vi "Init Device.vi"(8 "error in (no error)":errorcluster, 11 "Virtual Microscope in":refnum<class "Virtual Microscope.lvclass">) -> (0 "error out":errorcluster, 3 "Virtual Microscope out":refnum<class "Virtual Microscope.lvclass">)   [LabVIEW 2015, in "Virtual Microscope.lvlib" / "Virtual Microscope.lvclass"]
uses:
  Virtual Microscope.lvclass
  Virtual Microscope.lvclass/Virtual Microscope.ctl
  TE2000/TE2000.lvclass
  Eclipse TI/Eclipse TI.lvclass
  Device/Device.lvclass
  <vilib>/ActorFramework/Actor/Actor.lvclass
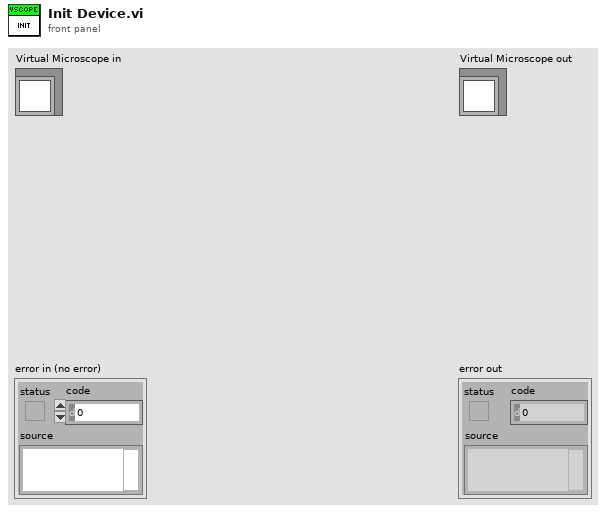
[diagram p1: front panel]
types:
  T1 = typedef "Microscope Configuration.ctl" = cluster{"Serial Port":refnum<visa-resource-name>, "Microscope Type":T2, "FilterBlockCassette1":refnum<k7>, "LightPathDrive":refnum<k7>, "INikonTI":refnum<k7>}
  T2 = typedef "Microscope Type.ctl" = enum16{"TE2000", "Eclipse Ti"}
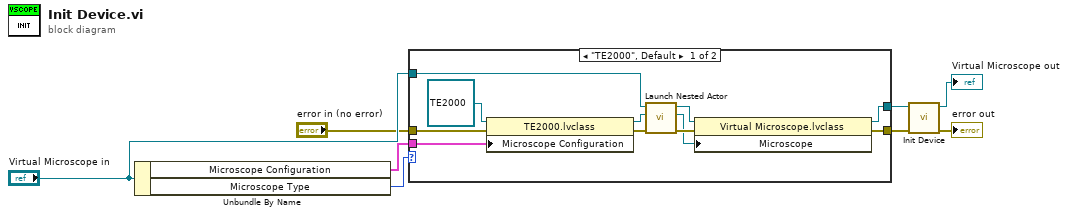
[diagram p0: block diagram]
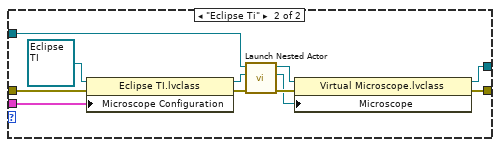
[diagram p2: hidden frame]
diagram:
  n1 = Unbundle By Name("Virtual Microscope in") -> ("Microscope Configuration"=w6:T1, "Microscope Type"=w5:T2)
  n2 = case shown="\"TE2000\", Default" w5 {
    tunnel: "Virtual Microscope in" -> [w18 w30]
    tunnel: [w12 w21] -> w1
    tunnel: w6 -> [w16 w28]
    tunnel: "error in (no error)" -> [w15 w27]
    tunnel: [w11 w23] -> w2
    frame "TE2000", Default {
      n3 = property class="TE2000.lvclass"(reference=refnum<class "TE2000.lvclass"> refnum ("TE2000.lvlib:TE2000.lvclass"), error in=w15, "Microscope Configuration"=w16) -> (reference out=w17:refnum<class "TE2000.lvclass">, error out=w14:errorcluster)
      n4 = call <vilib>:"Launch Nested Actor.vi"("error in (no error)"=w14, "Nested Actor"=w17, "Caller Actor in"=w18) -> ("error out"=w10:errorcluster, "Nested Actor's Enqueuer"=w9:refnum<class "Message Enqueuer.lvclass">, "Caller Actor out"=w13:refnum<class "Virtual Microscope.lvclass">)  [unwired: 6 in]
      n5 = property class="Virtual Microscope.lvclass"(reference=w13, error in=w10, "Microscope"=w9) -> (reference out=w12:refnum<class "Virtual Microscope.lvclass">, error out=w11:errorcluster)
    }
    frame "Eclipse Ti" {
      n6 = property class="Eclipse TI.lvclass"(reference=refnum<class "Eclipse TI.lvclass"> refnum ("Eclipse TI.lvlib:Eclipse TI.lvclass"), error in=w27, "Microscope Configuration"=w28) -> (reference out=w29:refnum<class "Eclipse TI.lvclass">, error out=w26:errorcluster)
      n7 = call <vilib>:"Launch Nested Actor.vi"("error in (no error)"=w26, "Nested Actor"=w29, "Caller Actor in"=w30) -> ("error out"=w24:errorcluster, "Nested Actor's Enqueuer"=w20:refnum<class "Message Enqueuer.lvclass">, "Caller Actor out"=w22:refnum<class "Virtual Microscope.lvclass">)  [unwired: 6 in]
      n8 = property class="Virtual Microscope.lvclass"(reference=w22, error in=w24, "Microscope"=w20) -> (reference out=w21:refnum<class "Virtual Microscope.lvclass">, error out=w23:errorcluster)
    }
  }
  n9 = call-parent "Init Device.vi"("error in (no error)"=w2, "Device in"=w1) -> ("error out"=→"error out":errorcluster, "Device out"=→"Virtual Microscope out":refnum<class "Virtual Microscope.lvclass">)  [unwired: 8 in]
